vi "Add Child.vi"(8 "error in (no error)":errorcluster, 10 "Child":refnum<data-value>, 11 "NodeRef In":refnum<data-value>) -> (0 "error out":errorcluster, 3 "NodeRef":refnum<data-value>)   [LabVIEW 2020, in "PicoG-ParserLexer.lvlib" / "Node.lvclass"]
doc: "Adds the <b>Child</b> node as the first child in the child list of the current node.\n\n<b>Error Codes:</b>\n<b>1556</b>: Nodes must be instantiated with Ctor first."
uses:
  Node.lvclass
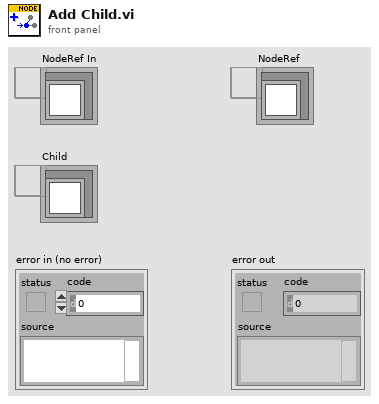
[diagram p1: front panel]
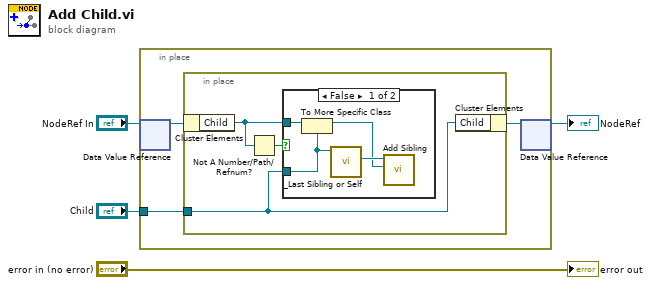
[diagram p0: block diagram]
diagram:
  n1 = in-place {
    in-place-border: "Child" -> [w6]
    n2 = in-place-dvr #1("NodeRef In") -> (w7:refnum<class "Node.lvclass">)  [unwired: 1 out]
    n3 = in-place {
      in-place-border: w6 -> [w8]
      n4 = in-place-cluster #2(w7) -> ("Child"=w9:refnum<data-value>)
      n5 = Not A Number/Path/Refnum?(number/path/refnum=w9) -> (NaN/Path/Refnum?=w10:bool)
      n6 = case shown="False" w10 {
        tunnel: w9 -> [w14 _]
        tunnel: w8 -> [w13 _]
        frame False {
          n7 = To More Specific Class(target class=w13, reference=w14) -> (specific class reference=w11:refnum<data-value>)  [unwired: 1 in, 1 out]
          n8 = call "_Last Sibling or Self.vi"("NodeRef In"=w13) -> ("Last Sibling or Self"=w12:refnum<data-value>)  [unwired: 8 in, 2 out]
          n9 = call "Add Sibling.vi"("Sibling"=w11, "NodeRef In"=w12) -> ()  [unwired: 8 in, 2 out]
        }
        frame True {
        }
      }
      n10 = in-place-cluster #2("Child"=w8) -> (w5:refnum<class "Node.lvclass">)
    }
    n11 = in-place-dvr #1(w5) -> (→"NodeRef":refnum<data-value>)  [unwired: 1 out]
  }
  "error out" <- "error in (no error)"
